vi "MANUAL FINAL.vi"() -> ()   [LabVIEW 2021]
uses:
  <vilib>/LabVIEW Interface for Arduino/LabVIEW Interface for Arduino.lvlib
panel:
  out "error out":errorcluster
  out "H":bool
  out "G":bool
  out "F":bool
  out "E":bool
  out "D":bool
  out "A":bool
  out "B":bool
  out "C":bool
  in  "delimiter":string="\t"
  in  "delimited string":string
  out "string array":string[](array[string])
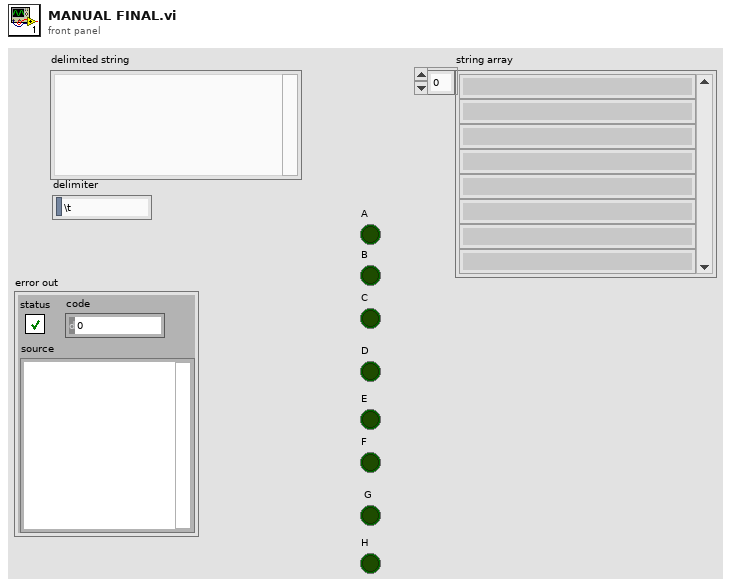
[diagram p1: front panel]
types:
  T1 = typedef "LabVIEW Interface for Arduino.lvlib/Arduino Resource.ctl" = cluster{"VISA resource":refnum<visa-resource-name>, "Board Type":T2, "Connection Type":enum8{"USB / Serial"}, "Bytes Per Packet (15)":u8}
  T2 = typedef "LabVIEW Interface for Arduino.lvlib/Board Type.ctl" = enum16{"Uno", "Dimuelanove w/Atmega 328", "Mega 2560"}
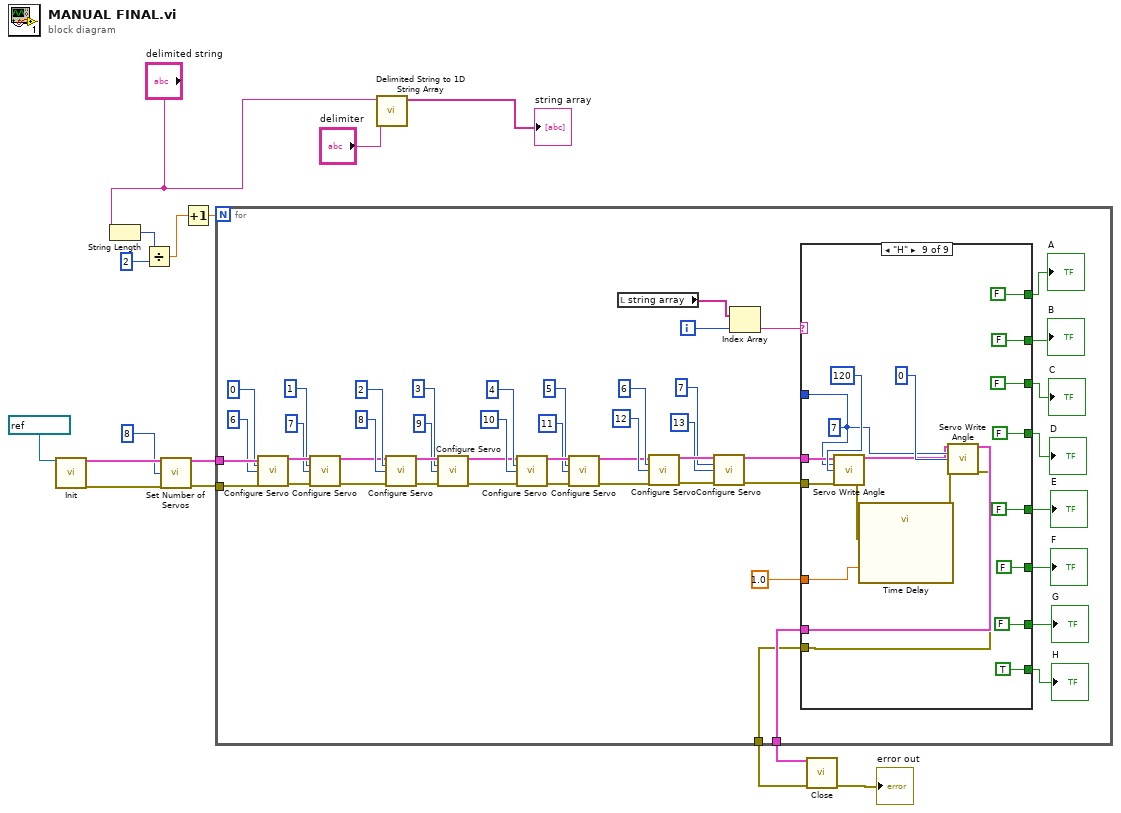
[diagram p0: block diagram]
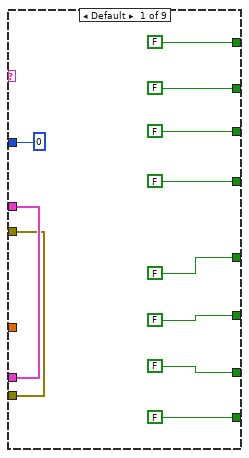
[diagram p2: hidden frame]
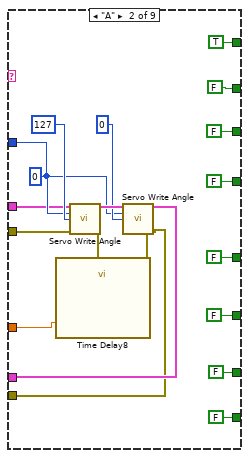
[diagram p3: hidden frame]
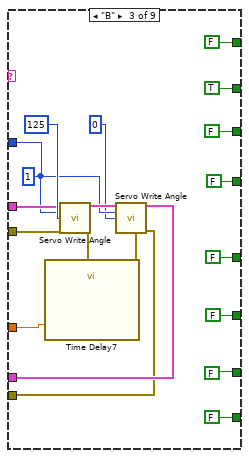
[diagram p4: hidden frame]
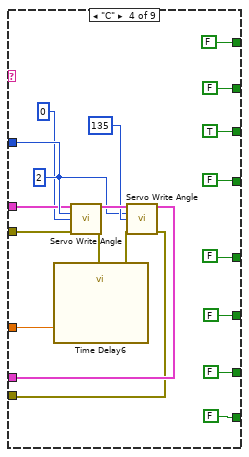
[diagram p5: hidden frame]
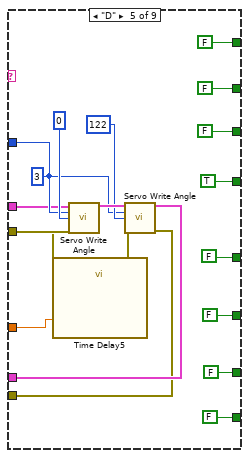
[diagram p6: hidden frame]
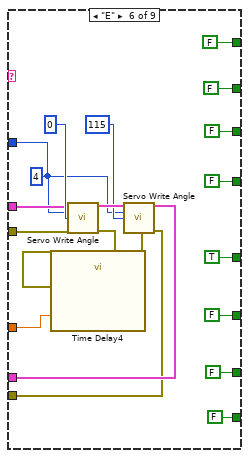
[diagram p7: hidden frame]
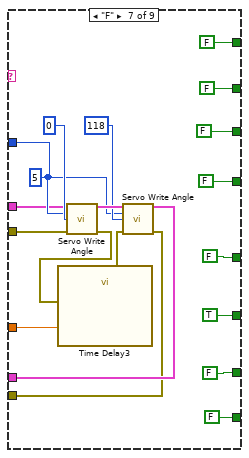
[diagram p8: hidden frame]
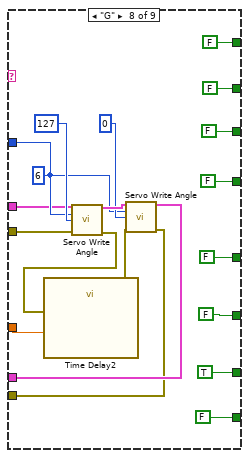
[diagram p9: hidden frame]
diagram:
  n1 = call <vilib>:"Init.vi"("VISA resource"=refnum<visa-resource-name> "COM3") -> ("Arduino Resource"=w12:T1, "error out"=w11:errorcluster)  [unwired: 17 in]
  n2 = String Length(string="delimited string") -> (length=w5:i32)
  n3 = Divide(x=w5, y=2) -> (x/y=w2:dbl)
  n4 = call <vilib>:"Set Number of Servos.vi"("Arduino Resource"=w12, "Number Of Servos (1)"=u8 8, "error in"=w11) -> ("Arduino Resource"=w10:T1, "error out"=w9:errorcluster)  [unwired: 11 in]
  n5 = Increment(x=w2) -> (x+1=w3:dbl)
  n6 = for {
    N: w3 -> [_]
    tunnel: w10 -> [w53]
    tunnel: w9 -> [w52]
    tunnel: [w45] -> w8
    tunnel: [w44] -> w7
    i -> [w64]
    n7 = call <vilib>:"Configure Servo.vi"("Arduino Resource"=w53, "Servo Number (0)"=u8 0, "DIO Pin (2)"=u8 6, "error in"=w52) -> ("Arduino Resource"=w50:T1, "error out"=w49:errorcluster)  [unwired: 10 in]
    n8 = call <vilib>:"Configure Servo.vi"("Arduino Resource"=w50, "Servo Number (0)"=u8 1, "DIO Pin (2)"=u8 7, "error in"=w49) -> ("Arduino Resource"=w25:T1, "error out"=w24:errorcluster)  [unwired: 10 in]
    n9 = call <vilib>:"Configure Servo.vi"("Arduino Resource"=w25, "Servo Number (0)"=u8 2, "DIO Pin (2)"=u8 8, "error in"=w24) -> ("Arduino Resource"=w42:T1, "error out"=w41:errorcluster)  [unwired: 10 in]
    n10 = call <vilib>:"Configure Servo.vi"("Arduino Resource"=w42, "Servo Number (0)"=u8 3, "DIO Pin (2)"=u8 9, "error in"=w41) -> ("Arduino Resource"=w23:T1, "error out"=w22:errorcluster)  [unwired: 10 in]
    n11 = call <vilib>:"Configure Servo.vi"("Arduino Resource"=w23, "Servo Number (0)"=u8 4, "DIO Pin (2)"=u8 10, "error in"=w22) -> ("Arduino Resource"=w36:T1, "error out"=w35:errorcluster)  [unwired: 10 in]
    n12 = call <vilib>:"Configure Servo.vi"("Arduino Resource"=w36, "Servo Number (0)"=u8 5, "DIO Pin (2)"=u8 11, "error in"=w35) -> ("Arduino Resource"=w21:T1, "error out"=w20:errorcluster)  [unwired: 10 in]
    n13 = local read "string array"() -> (w60:string[])
    n14 = call <vilib>:"Configure Servo.vi"("Arduino Resource"=w21, "Servo Number (0)"=u8 6, "DIO Pin (2)"=u8 12, "error in"=w20) -> ("Arduino Resource"=w30:T1, "error out"=w29:errorcluster)  [unwired: 10 in]
    n15 = call <vilib>:"Configure Servo.vi"("Arduino Resource"=w30, "Servo Number (0)"=u8 7, "DIO Pin (2)"=u8 13, "error in"=w29) -> ("Arduino Resource"=w18:T1, "error out"=w19:errorcluster)  [unwired: 10 in]
    n16 = Index Array(array=w60, index=w64) -> (element=w63:string)
    n17 = case shown="\"H\"" w63 {
      tunnel: [FALSE TRUE FALSE FALSE FALSE FALSE FALSE FALSE FALSE] -> w62
      tunnel: [FALSE FALSE TRUE FALSE FALSE FALSE FALSE FALSE FALSE] -> w54
      tunnel: [FALSE FALSE FALSE TRUE FALSE FALSE FALSE FALSE FALSE] -> w61
      tunnel: [FALSE FALSE FALSE FALSE TRUE FALSE FALSE FALSE FALSE] -> w59
      tunnel: [FALSE FALSE FALSE FALSE FALSE TRUE FALSE FALSE FALSE] -> w58
      tunnel: [FALSE FALSE FALSE FALSE FALSE FALSE TRUE FALSE FALSE] -> w57
      tunnel: [FALSE FALSE FALSE FALSE FALSE FALSE FALSE TRUE FALSE] -> w56
      tunnel: [FALSE FALSE FALSE FALSE FALSE FALSE FALSE FALSE TRUE] -> w55
      tunnel: [0 w83 w101 w122 w140 w157 w178 w197 w213] -> _
      tunnel: w18 -> [w66 w82 w104 w121 w139 w159 w177 w196 w217]
      tunnel: w19 -> [w65 w81 w103 w120 w138 w158 w176 w195 w216]
      tunnel: [w65 w79 w98 w118 w136 w155 w174 w193 w214] -> w44
      tunnel: [w66 w80 w99 w119 w137 w156 w175 w194 w215] -> w45
      tunnel: 1.0 ("Delay Time (s)") -> [_ w76 w95 w115 w133 w152 w171 w190 w209]
      frame Default {
      }
      frame "A" {
        w83 = u8 0 ("Servo Number")
        n18 = call <vilib>:"Servo Write Angle.vi"("Arduino Resource"=w82, "Servo Number"=w83, "Angle (Degrees)"=u8 127, "error in"=w81) -> ("Arduino Resource"=w85:T1, "error out"=w78:errorcluster)  [unwired: 10 in]
        n19 = call "Time Delay8"("error in (no error)"=w78, "Delay Time (s)"=w76) -> ("error out"=w77:errorcluster)  [unwired: 9 in]
        n20 = call <vilib>:"Servo Write Angle.vi"("Arduino Resource"=w85, "Servo Number"=w83, "Angle (Degrees)"=u8 0, "error in"=w77) -> ("Arduino Resource"=w80:T1, "error out"=w79:errorcluster)  [unwired: 10 in]
      }
      frame "B" {
        w101 = u8 1 ("Servo Number")
        n21 = call <vilib>:"Servo Write Angle.vi"("Arduino Resource"=w104, "Servo Number"=w101, "Angle (Degrees)"=u8 125, "error in"=w103) -> ("Arduino Resource"=w102:T1, "error out"=w97:errorcluster)  [unwired: 10 in]
        n22 = call "Time Delay7"("error in (no error)"=w97, "Delay Time (s)"=w95) -> ("error out"=w96:errorcluster)  [unwired: 9 in]
        n23 = call <vilib>:"Servo Write Angle.vi"("Arduino Resource"=w102, "Servo Number"=w101, "Angle (Degrees)"=u8 0, "error in"=w96) -> ("Arduino Resource"=w99:T1, "error out"=w98:errorcluster)  [unwired: 10 in]
      }
      frame "C" {
        w122 = u8 2 ("Servo Number")
        n24 = call <vilib>:"Servo Write Angle.vi"("Arduino Resource"=w121, "Servo Number"=w122, "Angle (Degrees)"=0, "error in"=w120) -> ("Arduino Resource"=w124:T1, "error out"=w117:errorcluster)  [unwired: 10 in]
        n25 = call "Time Delay6"("error in (no error)"=w117, "Delay Time (s)"=w115) -> ("error out"=w116:errorcluster)  [unwired: 9 in]
        n26 = call <vilib>:"Servo Write Angle.vi"("Arduino Resource"=w124, "Servo Number"=w122, "Angle (Degrees)"=u8 135, "error in"=w116) -> ("Arduino Resource"=w119:T1, "error out"=w118:errorcluster)  [unwired: 10 in]
      }
      frame "D" {
        w140 = u8 3 ("Servo Number")
        n27 = call <vilib>:"Servo Write Angle.vi"("Arduino Resource"=w139, "Servo Number"=w140, "Angle (Degrees)"=u8 0, "error in"=w138) -> ("Arduino Resource"=w142:T1, "error out"=w135:errorcluster)  [unwired: 10 in]
        n28 = call "Time Delay5"("error in (no error)"=w135, "Delay Time (s)"=w133) -> ("error out"=w134:errorcluster)  [unwired: 9 in]
        n29 = call <vilib>:"Servo Write Angle.vi"("Arduino Resource"=w142, "Servo Number"=w140, "Angle (Degrees)"=u8 122, "error in"=w134) -> ("Arduino Resource"=w137:T1, "error out"=w136:errorcluster)  [unwired: 10 in]
      }
      frame "E" {
        w157 = u8 4 ("Servo Number")
        n30 = call <vilib>:"Servo Write Angle.vi"("Arduino Resource"=w159, "Servo Number"=w157, "Angle (Degrees)"=u8 0, "error in"=w158) -> ("Arduino Resource"=w161:T1, "error out"=w154:errorcluster)  [unwired: 10 in]
        n31 = call "Time Delay4"("error in (no error)"=w154, "Delay Time (s)"=w152) -> ("error out"=w153:errorcluster)  [unwired: 9 in]
        n32 = call <vilib>:"Servo Write Angle.vi"("Arduino Resource"=w161, "Servo Number"=w157, "Angle (Degrees)"=u8 115, "error in"=w153) -> ("Arduino Resource"=w156:T1, "error out"=w155:errorcluster)  [unwired: 10 in]
      }
      frame "F" {
        w178 = u8 5 ("Servo Number")
        n33 = call <vilib>:"Servo Write Angle.vi"("Arduino Resource"=w177, "Servo Number"=w178, "Angle (Degrees)"=u8 0, "error in"=w176) -> ("Arduino Resource"=w180:T1, "error out"=w173:errorcluster)  [unwired: 10 in]
        n34 = call "Time Delay3"("error in (no error)"=w173, "Delay Time (s)"=w171) -> ("error out"=w172:errorcluster)  [unwired: 9 in]
        n35 = call <vilib>:"Servo Write Angle.vi"("Arduino Resource"=w180, "Servo Number"=w178, "Angle (Degrees)"=u8 118, "error in"=w172) -> ("Arduino Resource"=w175:T1, "error out"=w174:errorcluster)  [unwired: 10 in]
      }
      frame "G" {
        w197 = u8 6 ("Servo Number")
        n36 = call <vilib>:"Servo Write Angle.vi"("Arduino Resource"=w196, "Servo Number"=w197, "Angle (Degrees)"=u8 127, "error in"=w195) -> ("Arduino Resource"=w199:T1, "error out"=w192:errorcluster)  [unwired: 10 in]
        n37 = call "Time Delay2"("error in (no error)"=w192, "Delay Time (s)"=w190) -> ("error out"=w191:errorcluster)  [unwired: 9 in]
        n38 = call <vilib>:"Servo Write Angle.vi"("Arduino Resource"=w199, "Servo Number"=w197, "Angle (Degrees)"=u8 0, "error in"=w191) -> ("Arduino Resource"=w194:T1, "error out"=w193:errorcluster)  [unwired: 10 in]
      }
      frame "H" {
        w213 = u8 7 ("Servo Number")
        n39 = call <vilib>:"Servo Write Angle.vi"("Arduino Resource"=w217, "Servo Number"=w213, "Angle (Degrees)"=u8 120, "error in"=w216) -> ("Arduino Resource"=w212:T1, "error out"=w211:errorcluster)  [unwired: 10 in]
        n40 = call "Time Delay"("error in (no error)"=w211, "Delay Time (s)"=w209) -> ("error out"=w210:errorcluster)  [unwired: 9 in]
        n41 = call <vilib>:"Servo Write Angle.vi"("Arduino Resource"=w212, "Servo Number"=w213, "Angle (Degrees)"=u8 0, "error in"=w210) -> ("Arduino Resource"=w215:T1, "error out"=w214:errorcluster)  [unwired: 10 in]
      }
    }
    "A" <- w62
    "B" <- w54
    "C" <- w61
    "D" <- w59
    "E" <- w58
    "F" <- w57
    "G" <- w56
    "H" <- w55
  }
  n42 = call <vilib>:"Delimited String to 1D String Array.vi"("delimiter"="delimiter", "delimited string"="delimited string") -> ("string array"=→"string array":string[])  [unwired: 9 in]
  n43 = call <vilib>:"Close.vi"("Arduino Resource"=w8, "error in"=w7) -> ("error out"=→"error out":errorcluster)  [unwired: 13 in]
